vi "Read Values.vi"(11 "StepTypeMenuItem in":refnum<class "StepTypeMenuItem.lvclass">) -> (1 "Group":string, 2 "Display Name":string, 3 "Step Type":string)   [LabVIEW 2020, in "TSnax UI.lvlib" / "StepTypeMenuItem.lvclass"]
uses:
  StepTypeMenuItem.lvclass
  StepTypeMenuItem.lvclass/StepTypeMenuItem.ctl
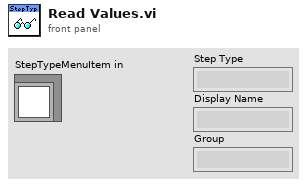
[diagram p1: front panel]
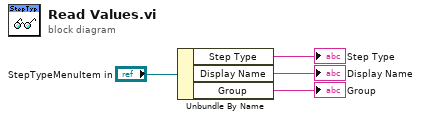
[diagram p0: block diagram]
diagram:
  n1 = Unbundle By Name("StepTypeMenuItem in") -> ("Step Type"=→"Step Type":string, "Display Name"=→"Display Name":string, "Group"=→"Group":string)
